vi "ALTS-2015 Write Robot Task.vi"(8 "error in (no error)":errorcluster, 11 "Task Details":T4) -> (0 "error out":errorcluster, 3 "Next State to Execute":T3=enum."Wait for Robot Availability", 5 "Last Robot Task":T2, 7 "Last Robot Task Out Station #":T1)   [LabVIEW 2013]
uses:
  Controls/ALTS-2015 Serial Details.ctl
  Controls/ALTS-2015 Station Cluster.ctl
  Controls/ALTS-2015 Serial DB Details.ctl
  Controls/ALTS-2015 Auto Program States.ctl
  Controls/ALTS-2015 Robot Tasks.ctl
  Controls/ALTS-2015 LV2GBL Station Info Options.ctl
  Controls/ALTS-2015 Station Details.ctl
  Controls/ALTS-2015 Status Ring Indicator.ctl
  Controls/ALTS-2015 Write Robot Task OPC Options.ctl
  Controls/ALTS-2015 Robot FIFO Queue Options.ctl
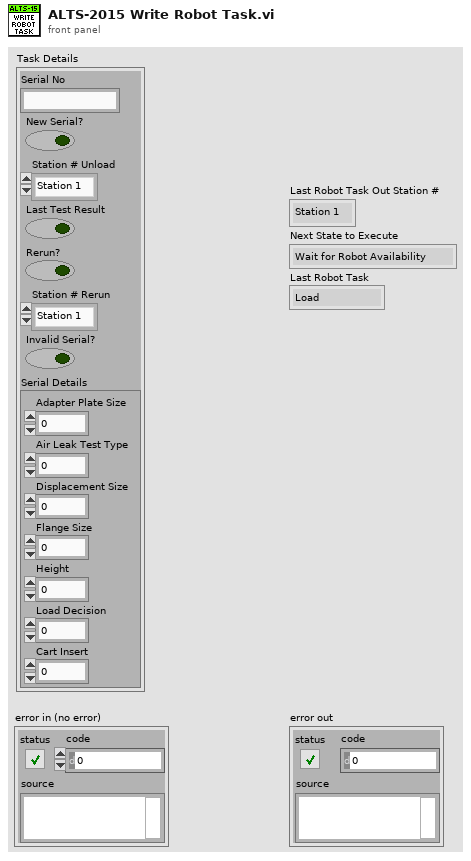
[diagram p1: front panel]
types:
  T1 = typedef "ALTS-2015 Station Cluster.ctl" = enum16{"Station 1", "Station 2", "Station 3", "Station 4"}
  T2 = typedef "ALTS-2015 Robot Tasks.ctl" = enum16{"Load", "Unload", "Rerun", "Invalid Serial"}
  T3 = typedef "ALTS-2015 Auto Program States.ctl" = enum16{"<------ Robot Handler States ------>", "Wait for Robot Availability", "Check Last Task by Robot", "Wait & Read Task from Queue", "Write New Task Details to Robot", "Write Task Available for Robot", "Check Robot for Unavailbilty", "Write Task Unavailable for Robot", "<------------ Other ------------>", "Error", "Exit"}
  T4 = typedef "ALTS-2015 Serial Details.ctl" = cluster{"Serial No":string, "New Serial?":bool, "Station # Unload":T1, "Last Test Result":bool, "Rerun?":bool, "Station # Rerun":T1, "Invalid Serial?":bool, "Serial Details":T5}
  T5 = typedef "ALTS-2015 Serial DB Details.ctl" = cluster{"Adapter Plate Size":i32, "Air Leak Test Type ":i32, "Displacement Size":i32, "Flange Size":i32, "Height":i32, "Load Decision":i32, "Cart Insert":i32}
  T6 = typedef "ALTS-2015 Station Details.ctl" = cluster{"Station Number":string, "Work Order Number":string, "Sensor Name":string, "Pressure (PSI)":string, "Flow (SCCM)":string, "Test Time ":string, "Test Result":string, "Serial Number":string, "Station Status":T7, "SW assigned UUT":bool, "Rerun Count":i32, "Test Type":i32, "Load Decision":i32}
  T7 = typedef "ALTS-2015 Status Ring Indicator.ctl" = u16
  T8 = typedef "ALTS-2015 LV2GBL Station Info Options.ctl" = enum16{"Init", "Read", "Read All", "Write Sensor ID", "Write  Work Order", "Write Serial Number", "Write Test Data", "Write Station Status", "Write Station Occupancy", "Write Station Test Type", "Write Rerun", "Write Load Decision", "Clear All", "Clear Test Result"}
  T9 = typedef "ALTS-2015 Write Robot Task OPC Options.ctl" = enum16{"Write New Serial Task", "Write Rerun Task", "Write Unload Task", "Write Invalid Serial Task"}
  T10 = typedef "ALTS-2015 Robot FIFO Queue Options.ctl" = enum16{"Init", "Enqueue", "Dequeue", "Get FIFO Elements", "Flush", "Destroy"}
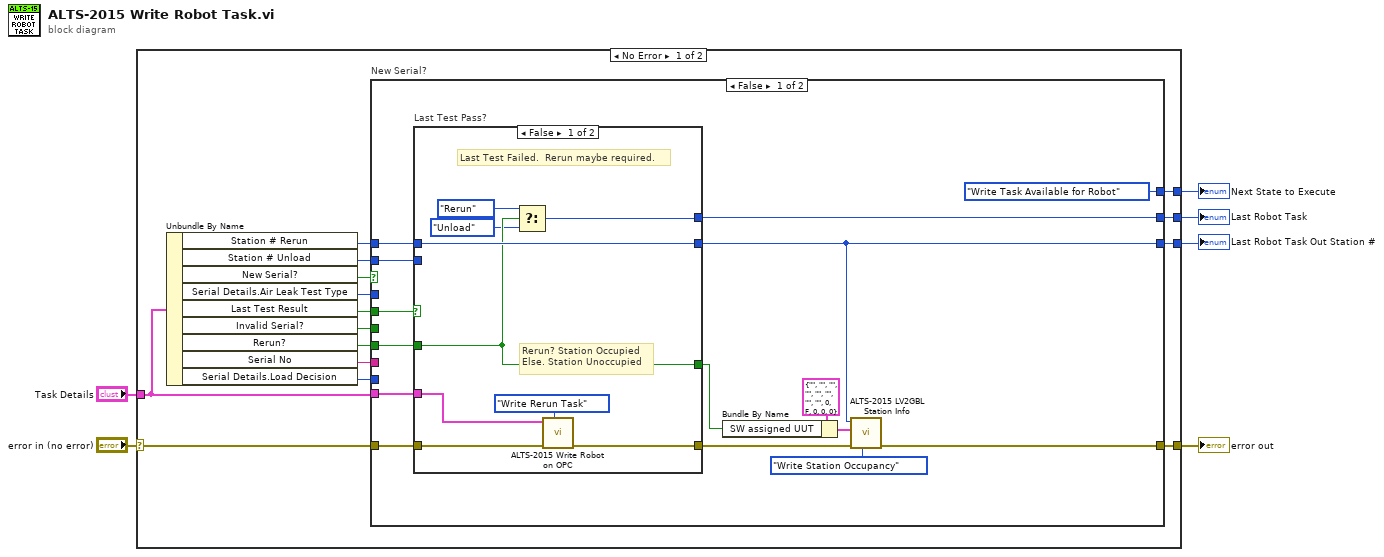
[diagram p0: block diagram]
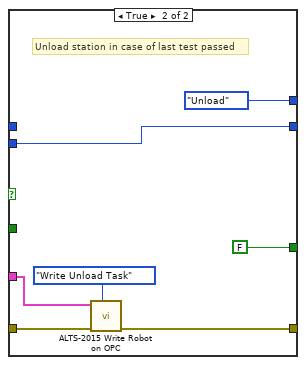
[diagram p2: hidden frame]
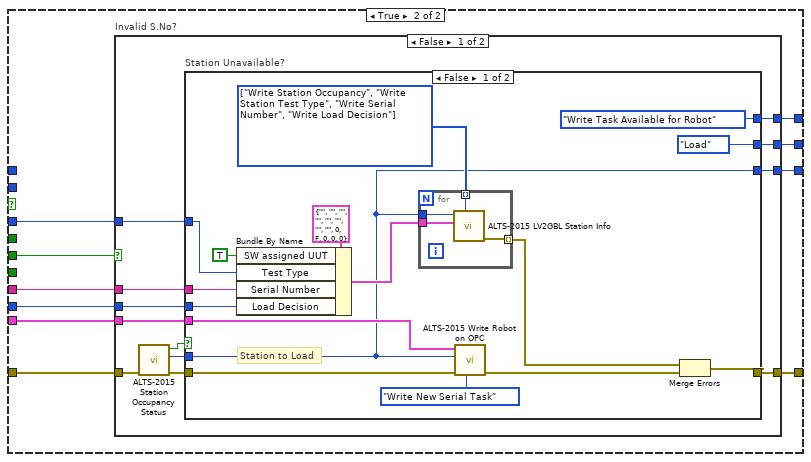
[diagram p3: hidden frame]
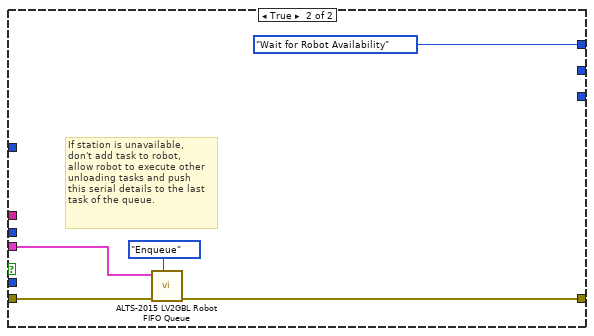
[diagram p4: hidden frame]
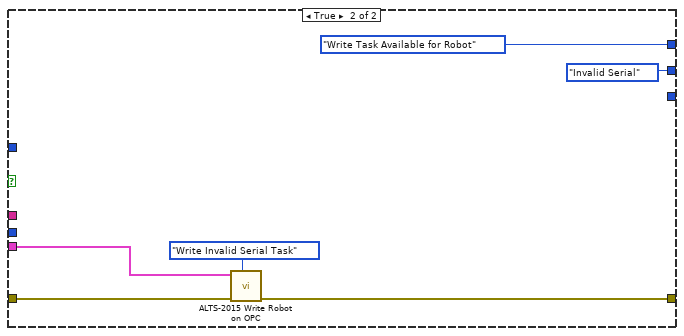
[diagram p5: hidden frame]
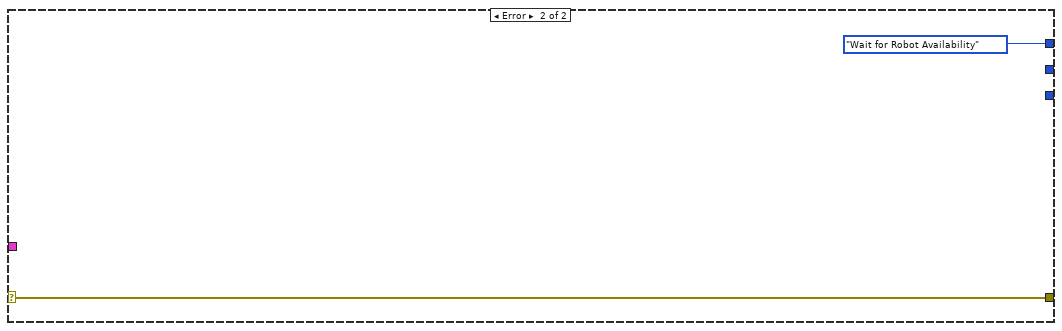
[diagram p6: hidden frame]
diagram:
  n1 = case shown="No Error" "error in (no error)" {
    selector: "error in (no error)" -> [w11 w107]
    tunnel: [w20 ALTS-2015_Auto_Program_States."Wait for Robot Availability"] -> w6
    tunnel: [w18 w107] -> w5
    tunnel: "Task Details" -> [w17 _]
    tunnel: [w8 _] -> w2
    tunnel: [w7 _] -> w1
    frame No Error {
      n2 = Unbundle By Name(w17) -> ("Station # Rerun"=w12:T1, "Station # Unload"=w13:T1, "New Serial?"=w19:bool, "Serial Details.Air Leak Test Type"=w16:i32, "Last Test Result"=w15:bool, "Invalid Serial?"=w21:bool, "Rerun?"=w14:bool, "Serial No"=w10:string, "Serial Details.Load Decision"=w9:i32)
      n3 = case "New Serial?" shown="False" w19 {
        tunnel: [ALTS-2015_Auto_Program_States."Write Task Available for Robot" w59] -> w20
        tunnel: [w23 w62] -> w18
        tunnel: w11 -> [w32 w61]
        tunnel: w17 -> [w30 w60]
        tunnel: w21 -> [_ w58]
        tunnel: w16 -> [_ w57]
        tunnel: w15 -> [w31 _]
        tunnel: w14 -> [w29 _]
        tunnel: w13 -> [w27 _]
        tunnel: w12 -> [w28 _]
        tunnel: w10 -> [_ w56]
        tunnel: w9 -> [_ w55]
        tunnel: [w26 w54] -> w8
        tunnel: [w25 w53] -> w7
        frame False {
          n4 = case "Last Test Pass?" shown="False" w31 {
            tunnel: [w40 FALSE ("Rerun?")] -> w24
            tunnel: w30 -> [w45 w49]
            tunnel: w32 -> [w44 w51]
            tunnel: [w43 w50] -> w22
            tunnel: w29 -> [w40 _]
            tunnel: [w41 w47] -> w25
            tunnel: w28 -> [w41 _]
            tunnel: w27 -> [_ w47]
            tunnel: [w37 ALTS-2015_Robot_Tasks."Unload" ("Last Robot Task")] -> w26
            frame False {
              # "Rerun? Station Occupied\nElse. Station Unoccupied"
              # "Last Test Failed.  Rerun maybe required."
              n5 = Select(t=ALTS-2015_Robot_Tasks."Rerun" ("Last Robot Task"), s=w40, f=ALTS-2015_Robot_Tasks."Unload" ("Last Robot Task")) -> (s? t:f=w37:T2)
              n6 = call "ALTS-2015 Write Robot on OPC.vi"("Option"=ALTS-2015_Write_Robot_Task_OPC_Options."Write Rerun Task", "error in (no error)"=w44, "Serial Details in"=w45) -> ("error out"=w43:errorcluster)  [unwired: 8 in]
            }
            frame True {
              # "Unload station in case of last test passed"
              n7 = call "ALTS-2015 Write Robot on OPC.vi"("Option"=ALTS-2015_Write_Robot_Task_OPC_Options."Write Unload Task", "error in (no error)"=w51, "Serial Details in"=w49) -> ("error out"=w50:errorcluster)  [unwired: 8 in]
            }
          }
          n8 = Bundle By Name(cluster=T6 {"Station Number"="", "Work Order Number"="", "Sensor Name"="", "Pressure (PSI)"="", "Flow (SCCM)"="", "Test Time "="", "Test Result"="", "Serial Number"="", "Station Status"=0, "SW assigned UUT"=FALSE, "Rerun Count"=0, "Test Type"=0, "Load Decision"=0} ("Station"), "SW assigned UUT"=w24) -> (w33:T6)
          n9 = call "ALTS-2015 LV2GBL Station Info.vi"("Options"=ALTS-2015_LV2GBL_Station_Info_Options."Write Station Occupancy", "error in"=w22, "Station"=w33, "Station Cluster"=w25) -> ("error out"=w23:errorcluster)  [unwired: 5 in, 2 out]
        }
        frame True {
          n10 = case "Invalid S.No?" shown="False" w58 {
            tunnel: [w72 w103] -> w62
            tunnel: w61 -> [w70 w104]
            tunnel: w60 -> [w69 w102]
            tunnel: [w68 ALTS-2015_Auto_Program_States."Write Task Available for Robot"] -> w59
            tunnel: w57 -> [w67 _]
            tunnel: w56 -> [w66 _]
            tunnel: w55 -> [w65 _]
            tunnel: [w64 ALTS-2015_Robot_Tasks."Invalid Serial" ("Last Robot Task")] -> w54
            tunnel: [w63 _] -> w53
            frame False {
              n11 = call "ALTS-2015 Station Occupancy Status.vi"("error in"=w70) -> ("error out"=w71:errorcluster, "Available Station"=w73:T1, "Station Unavailable"=w74:bool)  [unwired: 8 in]
              n12 = case "Station Unavailable?" shown="False" w74 {
                tunnel: w73 -> [w75 _]
                tunnel: [w79 w97] -> w72
                tunnel: w71 -> [w90 w98]
                tunnel: w69 -> [w85 w96]
                tunnel: [ALTS-2015_Auto_Program_States."Write Task Available for Robot" ALTS-2015_Auto_Program_States."Wait for Robot Availability"] -> w68
                tunnel: w67 -> [w83 _]
                tunnel: w66 -> [w82 _]
                tunnel: w65 -> [w80 _]
                tunnel: [ALTS-2015_Robot_Tasks."Load" ("Last Robot Task") _] -> w64
                tunnel: [w75 _] -> w63
                frame False {
                  w77 = T8[] [enum."Write Station Occupancy", enum."Write Station Test Type", enum."Write Serial Number", enum."Write Load Decision"] items=["Init", "Read", "Read All", "Write Sensor ID", "Write  Work Order", "Write Serial Number", "Write Test Data", "Write Station Status", "Write Station Occupancy", "Write Station Test Type", "Write Rerun", "Write Load Decision", "Clear All", "Clear Test Result"]
                  # "Station to Load"
                  n13 = Bundle By Name(cluster=T6 {"Station Number"="", "Work Order Number"="", "Sensor Name"="", "Pressure (PSI)"="", "Flow (SCCM)"="", "Test Time "="", "Test Result"="", "Serial Number"="", "Station Status"=0, "SW assigned UUT"=FALSE, "Rerun Count"=0, "Test Type"=0, "Load Decision"=0} ("Station"), "SW assigned UUT"=TRUE ("Rerun?"), "Test Type"=w83, "Serial Number"=w82, "Load Decision"=w80) -> (w81:T6)
                  n14 = for {
                    tunnel: w81 -> [w94]
                    tunnel: w75 -> [w93]
                    tunnel: [w92] -> w78 mode=indexing
                    tunnel: w77 -> [w91] mode=indexing
                    n15 = call "ALTS-2015 LV2GBL Station Info.vi"("Options"=w91, "Station"=w94, "Station Cluster"=w93) -> ("error out"=w92:errorcluster)  [unwired: 6 in, 2 out]
                  }
                  n16 = call "ALTS-2015 Write Robot on OPC.vi"("Option"=ALTS-2015_Write_Robot_Task_OPC_Options."Write New Serial Task", "error in (no error)"=w90, "Station # Load"=w75, "Serial Details in"=w85) -> ("error out"=w86:errorcluster)  [unwired: 7 in]
                  n17 = Merge Errors(w78, w86) -> (w79:errorcluster)
                }
                frame True {
                  # "If station is unavailable,\ndon't add task to robot,\nallow robot to execute other\nunloading tasks and push\nthis serial details to the last\ntask of the queue."
                  n18 = call "ALTS-2015 LV2GBL Robot FIFO Queue.vi"("Options"=ALTS-2015_Robot_FIFO_Queue_Options."Enqueue" ("Enum"), "error in (no error)"=w98, "Task Details In"=w96) -> ("error out"=w97:errorcluster)  [unwired: 4 in, 4 out]
                }
              }
            }
            frame True {
              n19 = call "ALTS-2015 Write Robot on OPC.vi"("Option"=ALTS-2015_Write_Robot_Task_OPC_Options."Write Invalid Serial Task", "error in (no error)"=w104, "Serial Details in"=w102) -> ("error out"=w103:errorcluster)  [unwired: 8 in]
            }
          }
        }
      }
    }
    frame Error {
    }
  }
  "Next State to Execute" <- w6
  "error out" <- w5
  "Last Robot Task" <- w2
  "Last Robot Task Out Station #" <- w1
